vi "MBUS_FGV_ConnectionRef.vi"(10 "ConnectionRefIn":T1, 11 "CMD":enum16{"GET", "SET"}(ring)) -> (0 "error out":errorcluster, 2 "ConnectionRefOut":T1)   [LabVIEW 2012, in "MBUS_Modbus.lvlib"]
uses:
  MBUS_Modbus.lvlib
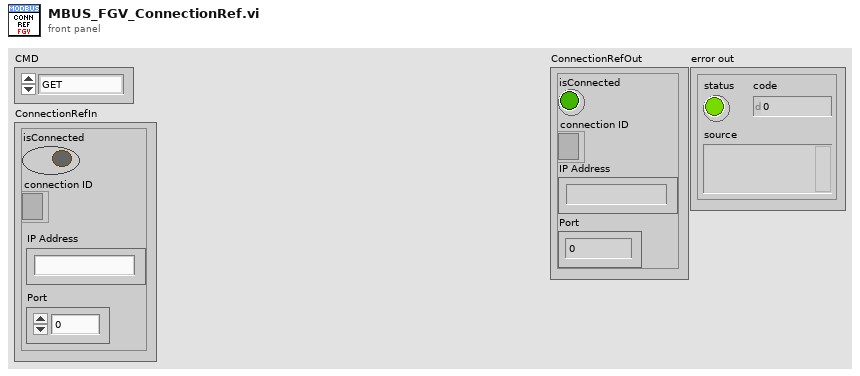
[diagram p1: front panel]
types:
  T1 = cluster{"isConnected":bool, "connection ID":refnum<k5>, "IP Address":string, "Port":dbl}
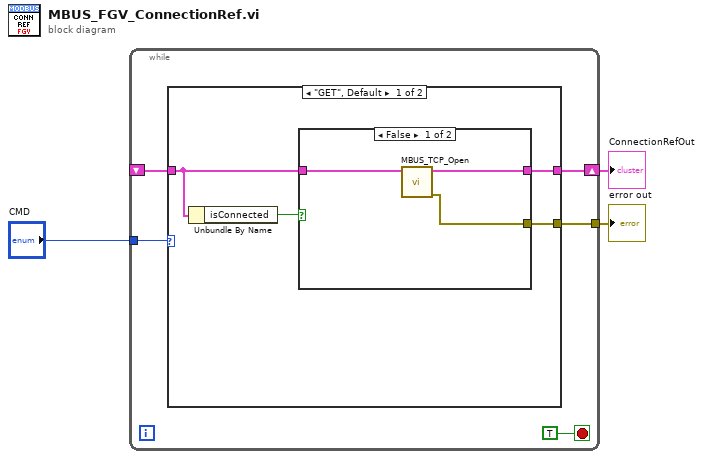
[diagram p0: block diagram]
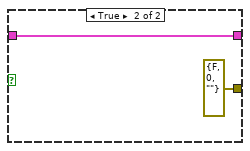
[diagram p2: hidden frame]
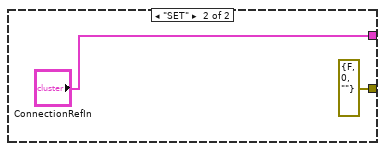
[diagram p3: hidden frame]
diagram:
  n1 = while {
    tunnel: "CMD" -> [w7]
    shift-right: [w5] -> w2
    shift-left: _ -> [w6]
    tunnel: [w4] -> w1
    stop <- TRUE stop-if-true
    n2 = case shown="\"GET\", Default" w7 {
      tunnel: w6 -> [w11 _]
      tunnel: [w10 "ConnectionRefIn"] -> w5
      tunnel: [w9 errorcluster {"status"=FALSE, "code"=0, "source"=""} ("error out")] -> w4
      frame "GET", Default {
        n3 = Unbundle By Name(w11) -> ("isConnected"=w12:bool)
        n4 = case shown="False" w12 {
          tunnel: w11 -> [w15 w17]
          tunnel: [w14 w17] -> w10
          tunnel: [w13 errorcluster {"status"=FALSE, "code"=0, "source"=""} ("error out")] -> w9
          frame False {
            n5 = call "MBUS_TCP_Open.vi"("ConnectionRefIn in"=w15) -> ("error out"=w13:errorcluster, "ConnectionRefIn out"=w14:T1)  [unwired: 9 in]
          }
          frame True {
          }
        }
      }
      frame "SET" {
      }
    }
  }
  "ConnectionRefOut" <- w2
  "error out" <- w1
